vi "Trumpf_RD_DataBaseUpload_AutoReport1.vi"(2 "error in (no error)":errorcluster, 3 "Bar_LIV_Data":path=path "D:/LabVIEW_prog/Trumpf_Database_Connect/TestData/Averaging_DM17-20_Post.xlsx") -> (0 "error out":errorcluster)   [LabVIEW 2017]
doc: "This example allows you to perform several tasks on the specified table in a database named LabVIEW.mdb located in the LabVIEW examples>>database directory.\n\nThis VI is running when you open it. Select one of the tabs and enter the appropriate data. Press the Go button to complete the displayed tab option.\n\nAutomatic - This option inserts a new record into the specified table. The record is specified by a cluster containing the correct number of elements and of the data types defined by the specified table. \n\nSQL Query - This option performs the specified SQL query.\n\nParameterized SQL Query - This option performs the specified SQL query as a parameterized SQL Query. This method is faster and more efficient than directly executing an SQL query because it sets up all the parameters prior to doing the command."
uses:
  <vilib>/addons/database/Connection.llb/DB Tools Open Connec (String).vi
  <vilib>/addons/database/Connection.llb/Conn Execute.vi
  <vilib>/addons/database/Recordset.llb/Rec Destroy - Connection.vi
  <vilib>/addons/database/NI_Database_API.lvlib
panel:
  out "Written Bar LIV Data":T1(array[cluster])
  out "Database Column":string[](array[string])
  # "Overview: Demonstrates how to insert records into databases, and perform SQL queries.\nRequirements: Database Connectivity Toolkit\nInstructions:\nRun the VI."
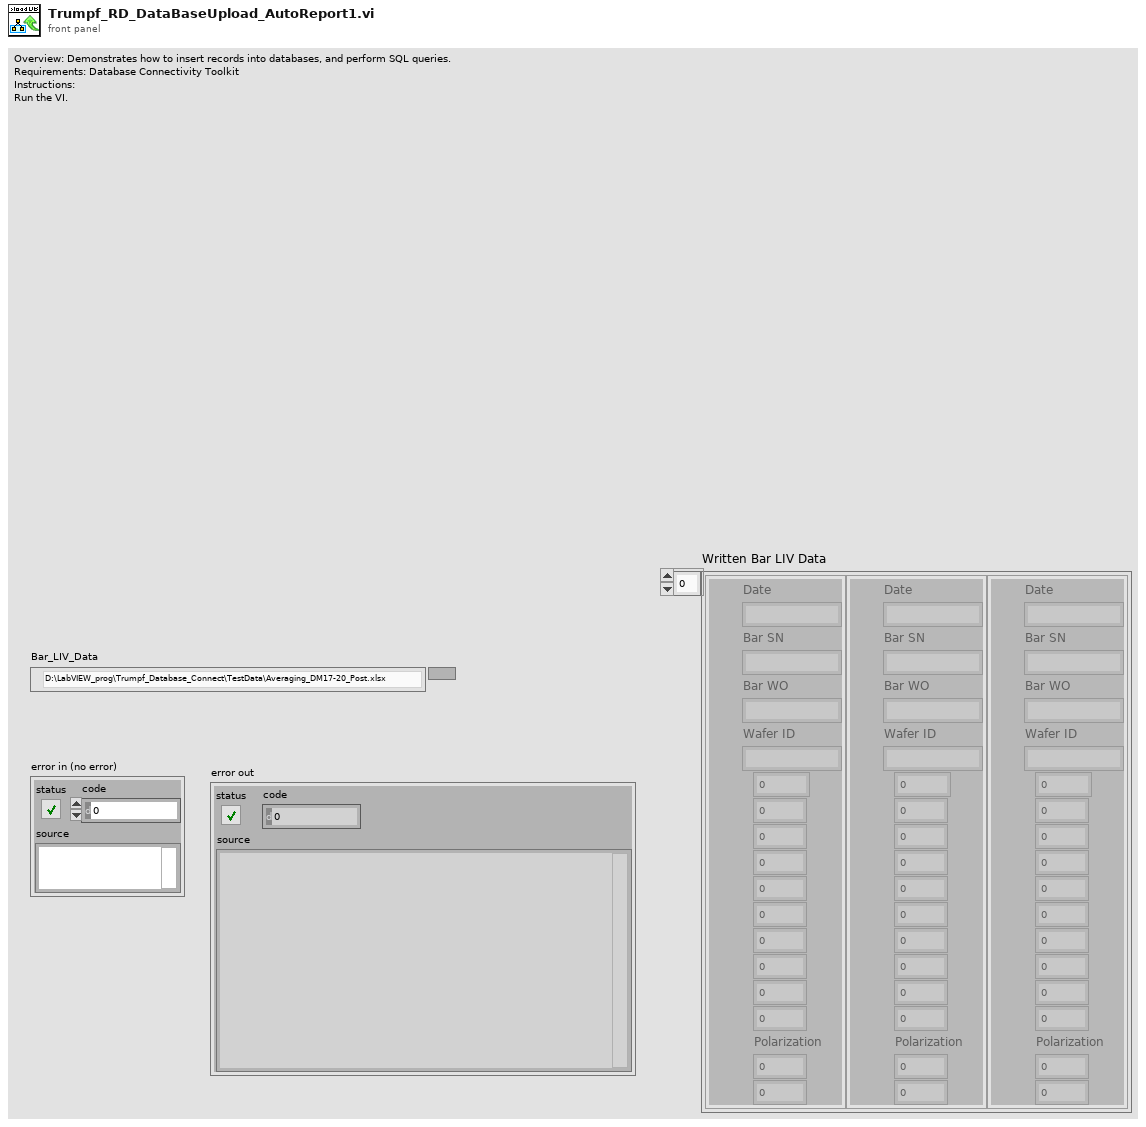
[diagram p1: front panel]
types:
  T1 = cluster{"Date":string, "Bar SN":string, "Bar WO":string, "Wafer ID":string, dbl, dbl, dbl, dbl, dbl, dbl, dbl, dbl, dbl, dbl, "Polarization":dbl, dbl}[]
  T2 = cluster{"Date":string, "LIV Data":dbl[][], "Polarization":dbl, "Bar SN":string, "Bar WO":string, "Wafer ID":string}
  T3 = typedef "NI_Database_API.lvlib/Conn ObjectReference.ctl" = refnum<k1>
  T4 = cluster{"Date":string, "Bar SN":string, "Bar WO":string, "Wafer ID":string, dbl, dbl, dbl, dbl, dbl, dbl, dbl, dbl, dbl, dbl, "Polarization":dbl, dbl}
  T5 = typedef "NI_Database_API.lvlib/Rec ObjectReference.ctl" = refnum<k1>
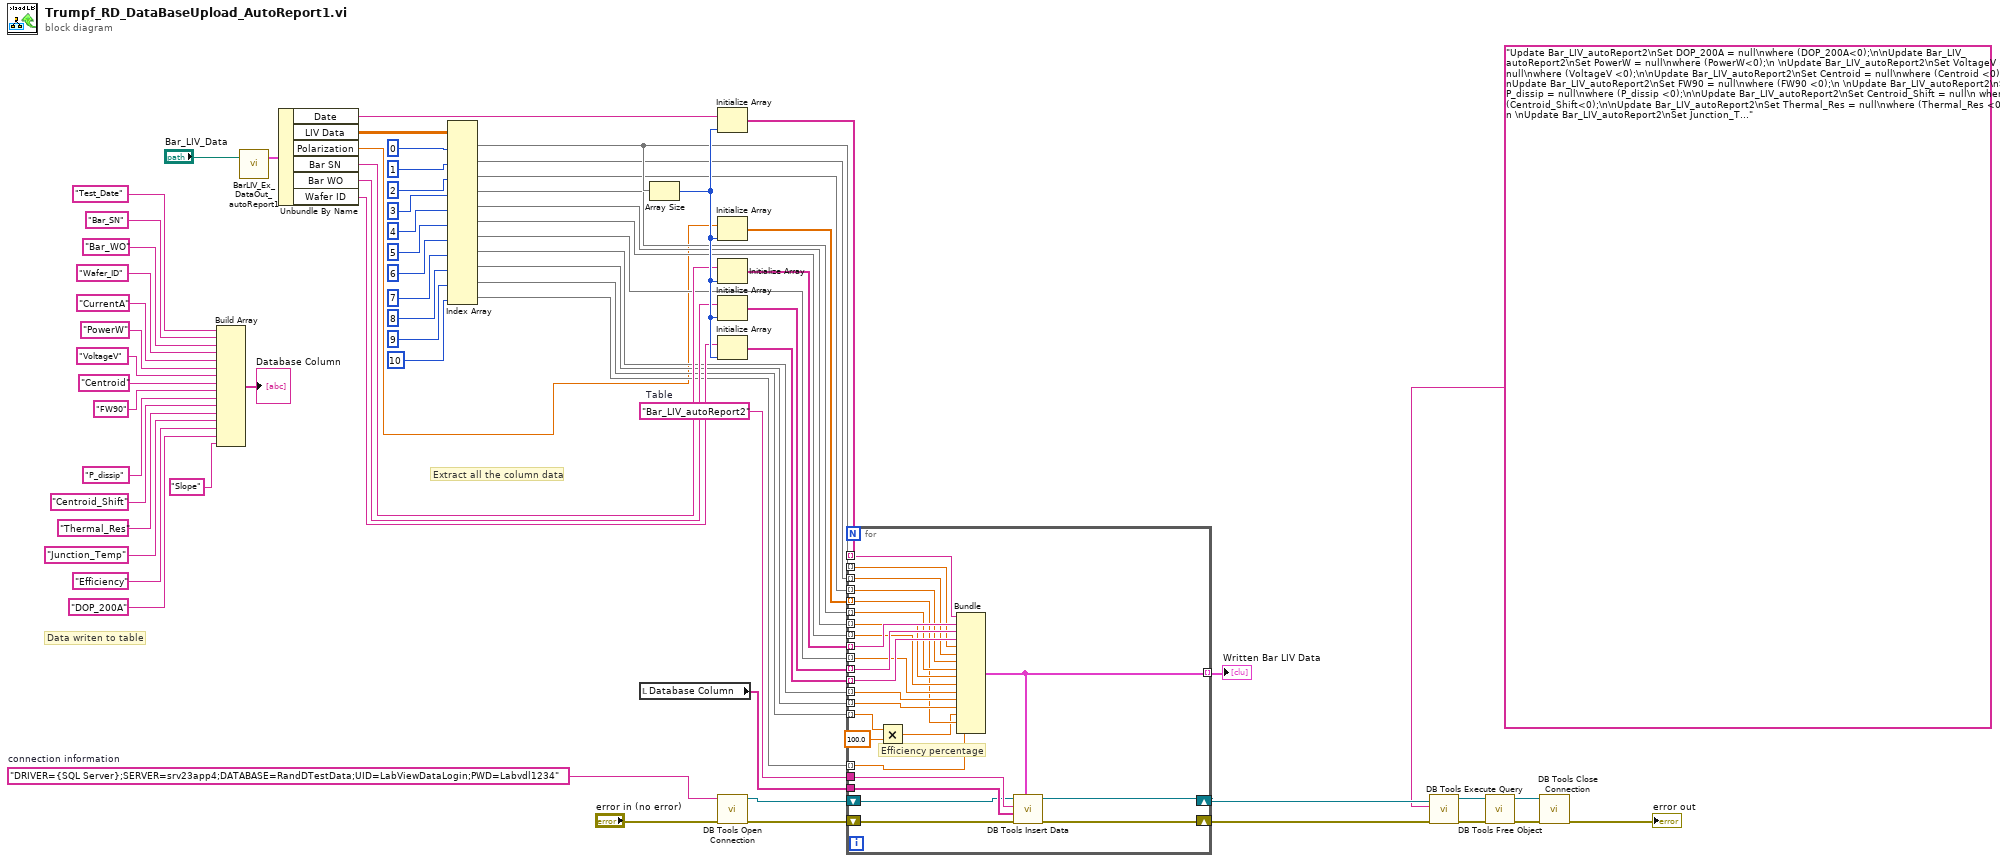
[diagram p0: block diagram]
diagram:
  w8 = "Bar_LIV_autoReport2"  # Table
  w63 = "DRIVER={SQL Server};SERVER=srv23app4;DATABASE=RandDTestData;UID=LabViewDataLogin;PWD=Labvdl1234"  # connection information
  # "Data writen to table"
  # "Extract all the column data"
  n1 = Build Array("Test_Date", "Bar_SN", "Bar_WO", "Wafer_ID", "CurrentA", "PowerW", "VoltageV", "Centroid", "FW90", "P_dissip", "Centroid_Shift", "Thermal_Res", "Junction_Temp", "Efficiency", "DOP_200A", "Slope") -> (→"Database Column":string[])
  n2 = call "BarLIV_Ex_DataOut_autoReport1.vi"("Bar_LIV_AutoRep"="Bar_LIV_Data") -> ("BarLIV AutoRep Output"=w59:T2)  [unwired: 1 in, 1 out]
  n3 = Unbundle By Name(w59) -> ("Date"=w34:string, "LIV Data"=w10:dbl[][], "Polarization"=w9:dbl, "Bar SN"=w33:string, "Bar WO"=w32:string, "Wafer ID"=w31:string)
  n4 = Index Array(array=w10, index (col) #1=0 ("disabled index (col)"), index (col) #2=1 ("index (col)"), index (col) #3=2 ("index (col)"), index (col) #4=3 ("index (col)"), index (col) #5=4 ("index (col)"), index (col) #6=5 ("index (col)"), index (col) #7=6 ("index (col)"), index (col) #8=7 ("index (col)"), index (col) #9=8 ("index (col)"), index (col) #10=9 ("index (col)"), index (col) #11=10 ("index (col)")) -> (element #1=w26:dbl[], element #2=w24:dbl[], element #3=w25:dbl[], element #4=w23:dbl[], element #5=w22:dbl[], element #6=w21:dbl[], element #7=w20:dbl[], element #8=w19:dbl[], element #9=w18:dbl[], element #10=w11:dbl[], element #11=w17:dbl[])  [unwired: 11 in]
  n5 = local read "Database Column"() -> (w15:string[])
  n6 = Array Size(array=w26) -> (size(s)=w35:i32)
  n7 = Initialize Array(w34, w35) -> (w30:string[])
  n8 = Initialize Array(w9, w35) -> (w16:dbl[])
  n9 = Initialize Array(w33, w35) -> (w29:string[])
  n10 = Initialize Array(w32, w35) -> (w28:string[])
  n11 = Initialize Array(w31, w35) -> (w27:string[])
  n12 = call-poly <vilib>:"DB Tools Open Connection.vi"("error in (no error)"="error in (no error)", "connection information"=w63) -> ("error out"=w14:errorcluster, "connection reference"=w13:T3)  [unwired: 6 in]
  n13 = for {
    tunnel: w30 -> [w93] mode=indexing
    tunnel: w29 -> [w92] mode=indexing
    tunnel: w28 -> [w91] mode=indexing
    tunnel: w27 -> [w90] mode=indexing
    tunnel: w26 -> [w89] mode=indexing
    tunnel: w25 -> [w87] mode=indexing
    tunnel: w24 -> [w88] mode=indexing
    tunnel: w23 -> [w86] mode=indexing
    tunnel: w22 -> [w85] mode=indexing
    tunnel: w21 -> [w84] mode=indexing
    tunnel: w20 -> [w83] mode=indexing
    tunnel: w19 -> [w82] mode=indexing
    tunnel: w18 -> [w81] mode=indexing
    tunnel: w11 -> [w71] mode=indexing
    tunnel: w16 -> [w80] mode=indexing
    tunnel: w17 -> [w79] mode=indexing
    tunnel: w8 -> [w78]
    tunnel: w15 -> [w77]
    shift-right: [w75] -> w7
    shift-left: w14 -> [w76]
    shift-right: [w74] -> w6
    shift-left: w13 -> [w73]
    tunnel: [w72] -> w12 mode=indexing
    # "Efficiency percentage"
    n14 = Multiply(x=w71, y=100.0) -> (x*y=w70:dbl)
    n15 = Bundle("Date"=w93, "Bar SN"=w92, "Bar WO"=w91, "Wafer ID"=w90, w89, w88, w87, w86, w85, w84, w83, w82, w81, w70, "Polarization"=w80, w79) -> (w72:T4)  [unwired: 1 in]
    n16 = call <vilib>:"DB Tools Insert Data.vi"("data"=w72, "error in (no error)"=w76, "columns"=w77, "table"=w78, "connection reference"=w73) -> ("error out"=w75:errorcluster, "connection reference out"=w74:T3)  [unwired: 5 in]
  }
  "Written Bar LIV Data" <- w12
  n17 = call-poly <vilib>:"DB Tools Execute Query.vi"("error in (no error)"=w7, "SQL query"="Update Bar_LIV_autoReport2\nSet DOP_200A = null\nwhere (DOP_200A<0);\n\nUpdate Bar_LIV_autoReport2\nSet PowerW = null\nwhere (PowerW<0);\n \nUpdate Bar_LIV_autoReport2\nSet VoltageV = null\nwhere (VoltageV <0);\n\nUpdate Bar_LIV_autoReport2\nSet Centroid = null\nwhere (Centroid <0);\n\nUpdate Bar_LIV_autoReport2\nSet FW90 = null\nwhere (FW90 <0);\n \nUpdate Bar_LIV_autoReport2\nSet P_dissip = null\nwhere (P_dissip <0);\n\nUpdate Bar_LIV_autoReport2\nSet Centroid_Shift = null\n where (Centroid_Shift<0);\n\nUpdate Bar_LIV_autoReport2\nSet Thermal_Res = null\nwhere (Thermal_Res <0);\n \nUpdate Bar_LIV_autoReport2\nSet Junction_Temp = null\nwhere (Junction_Temp <0);\n \nUpdate Bar_LIV_autoReport2\nSet Efficiency = null\nwhere (Efficiency<0);\n\nUpdate Bar_LIV_autoReport2\nSet DOP_200A = null \nwhere (DOP_200A<0);\n\nUpdate Bar_LIV_autoReport2\nSet Slope = null\n where (Slope<0);\n", "connection reference"=w6) -> ("error out"=w3:errorcluster, "recordset reference"=w5:T5)  [unwired: 5 in]
  n18 = call-poly <vilib>:"DB Tools Free Object.vi"("error in (no error)"=w3, "recordset reference"=w5) -> ("error out"=w2:errorcluster, "connection reference"=w4:T3)  [unwired: 8 in]
  n19 = call <vilib>:"DB Tools Close Connection.vi"("error in (no error)"=w2, "connection reference"=w4) -> ("error out"=→"error out":errorcluster)  [unwired: 5 in]
